vi "path_left.vi"() -> ()   [LabVIEW 2019]
uses:
  WSCbot_V3_Toolkit.lvlibp
panel:
  in  "get screw\n(XYZ) 2":cluster{"X":dbl, "Y":dbl, "Z":dbl}[](array[cluster])=[{"X"=0.0, "Y"=30.0, "Z"=0.0}, {"X"=0.0, "Y"=-30.0, "Z"=0.0}, {"X"=0.0, "Y"=0.0, "Z"=0.0}]
  in  "Stop Button 2":bool
  in  "Go home\n(XYZ)":cluster{"X":dbl, "Y":dbl, "Z":dbl}[](array[cluster])=[{"X"=0.0, "Y"=-296.0, "Z"=0.0}]
  in  "To stage\n(XYZ)":cluster{"X":dbl, "Y":dbl, "Z":dbl}[](array[cluster])=[{"X"=0.0, "Y"=-174.0, "Z"=0.0}, {"X"=143.0, "Y"=0.0, "Z"=0.0}, {"X"=0.0, "Y"=262.0, "Z"=0.0}]
  in  "get nut\nXYZ":cluster{"X":dbl, "Y":dbl, "Z":dbl}[](array[cluster])=[{"X"=0.0, "Y"=116.0, "Z"=0.0}]
  in  "cross hill\nXYZ":cluster{"X":dbl, "Y":dbl, "Z":dbl}[](array[cluster])=[{"X"=-70.0, "Y"=0.0, "Z"=0.0}, {"X"=0.0, "Y"=-145.0, "Z"=0.0}, {"X"=-77.0, "Y"=0.0, "Z"=0.0}]
  in  "to hill\n(XYZ)":cluster{"X":dbl, "Y":dbl, "Z":dbl}[](array[cluster])=[{"X"=122.0, "Y"=0.0, "Z"=0.0}, {"X"=0.0, "Y"=-60.0, "Z"=0.0}]
  in  "get screw\n(XYZ)":cluster{"X":dbl, "Y":dbl, "Z":dbl}[](array[cluster])=[{"X"=-125.0, "Y"=0.0, "Z"=0.0}, {"X"=0.0, "Y"=0.0, "Z"=0.0}, {"X"=0.0, "Y"=0.0, "Z"=0.0}]
  in  "To stage\n(XYZ)":cluster{"X":dbl, "Y":dbl, "Z":dbl}[](array[cluster])=[{"X"=66.0, "Y"=0.0, "Z"=0.0}, {"X"=0.0, "Y"=152.0, "Z"=0.0}, {"X"=70.0, "Y"=0.0, "Z"=0.0}, {"X"=0.0, "Y"=60.0, "Z"=0.0}]
  in  "To hill\n(XYZ)":cluster{"X":dbl, "Y":dbl, "Z":dbl}[](array[cluster])=[{"X"=0.0, "Y"=-106.0, "Z"=0.0}]
  in  "get nut\n(XYZ)":cluster{"X":dbl, "Y":dbl, "Z":dbl}[](array[cluster])=[{"X"=0.0, "Y"=-178.0, "Z"=-180.0}]
  in  "see mark & get screw\n(XYZ)":cluster{"X":dbl, "Y":dbl, "Z":dbl}[](array[cluster])=[{"X"=-26.0, "Y"=25.0, "Z"=0.0}, {"X"=0.0, "Y"=0.0, "Z"=-45.0}, {"X"=0.0, "Y"=0.0, "Z"=-45.0}, {"X"=0.0, "Y"=75.0, "Z"=-90.0}, {"X"=45.0, "Y"=0.0, "Z"=0.0}]
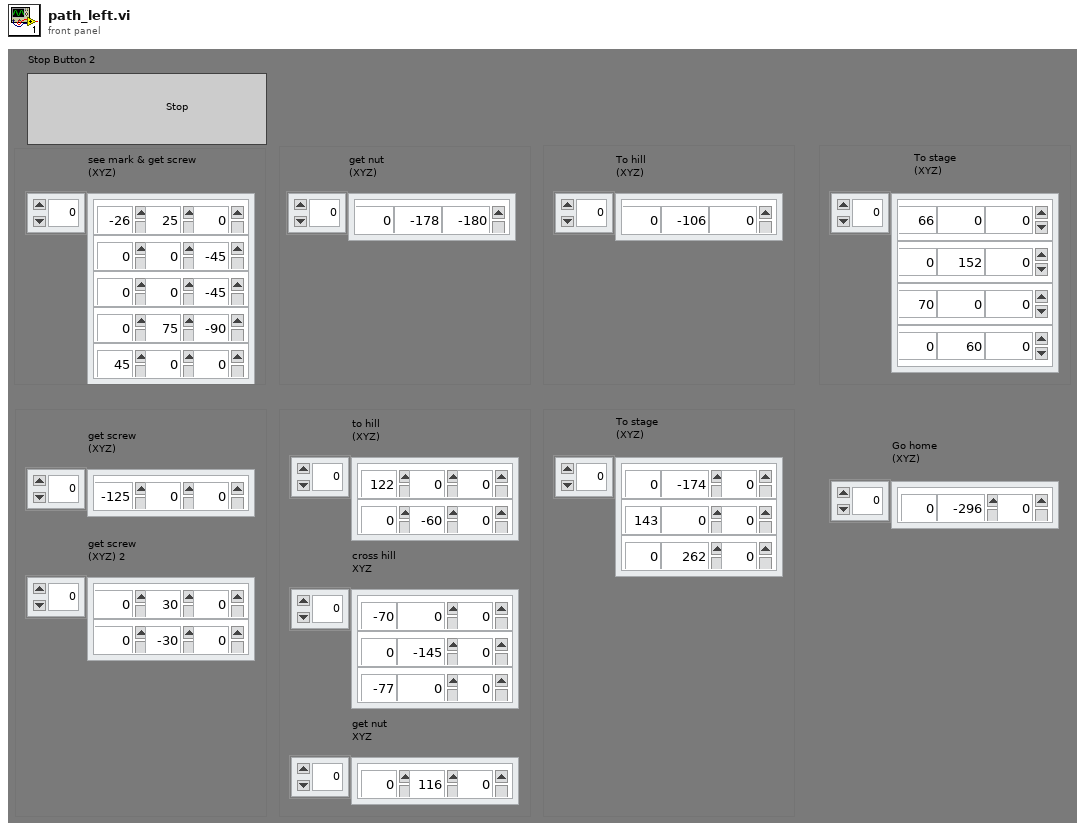
[diagram p1: front panel]
types:
  T1 = enum16{"Right_up", "Right_down", "Left_down", "Left_up", "left", "right", "up", "down"}
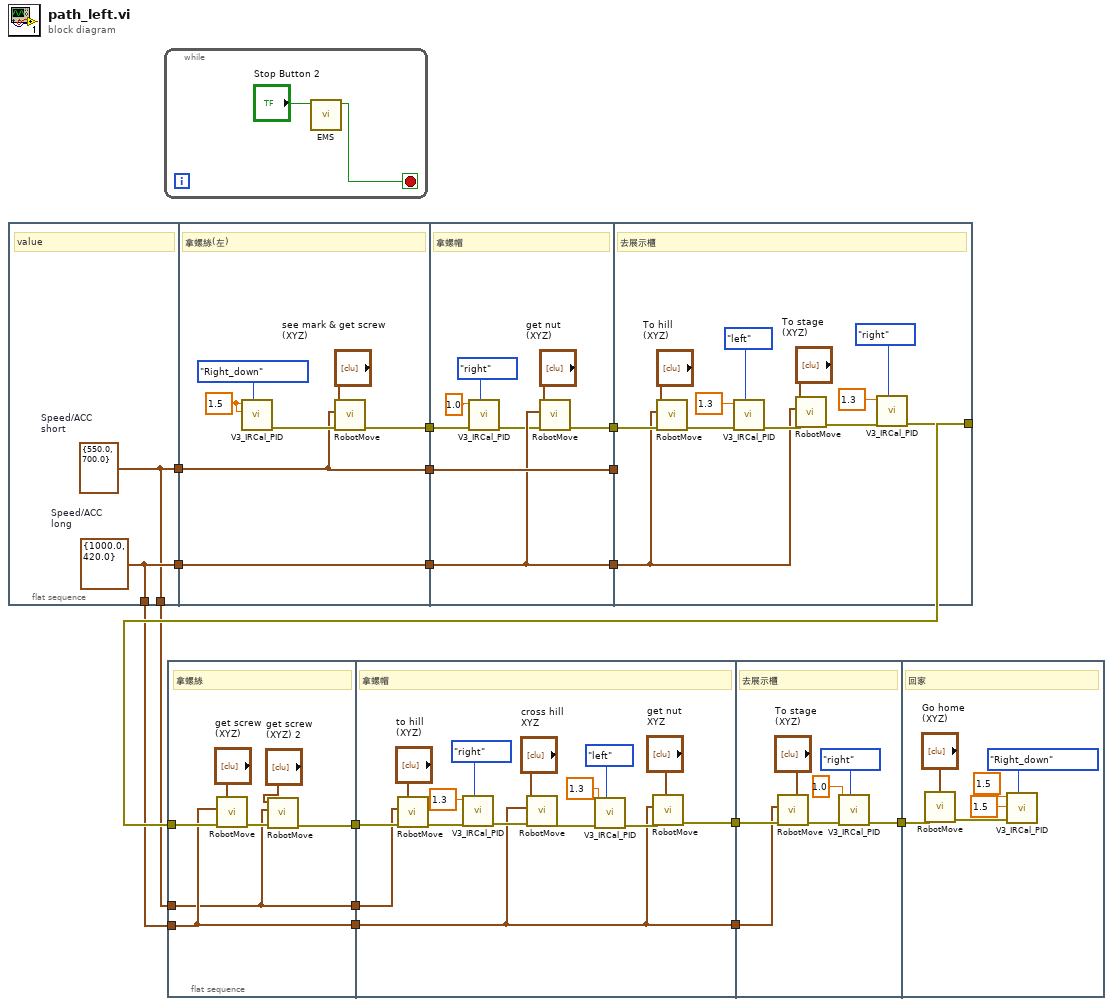
[diagram p0: block diagram]
diagram:
  n1 = flat-sequence {
    tunnel: [w18] -> w17
    tunnel: [w19] -> w10
    tunnel: [w19] -> w8
    tunnel: [w18] -> w7
    tunnel: w17 -> [w23]
    tunnel: [w24] -> w16
    tunnel: [w23] -> w14
    tunnel: [w22] -> w11
    tunnel: w10 -> [w22]
    tunnel: w16 -> [w30]
    tunnel: [w33] -> w15
    tunnel: w14 -> [w32]
    tunnel: [w32] -> w13
    tunnel: [w31] -> w12
    tunnel: w11 -> [w31]
    tunnel: w15 -> [w45]
    tunnel: w13 -> [_]
    tunnel: w12 -> [w39]
    tunnel: [w35] -> w9
    frame #0 {
      w18 = cluster{dbl, dbl} {550.0, 700.0}  # Speed/ACC short
      w19 = cluster{dbl, dbl} {1000.0, 420.0}  # Speed/ACC long
      # "value"
    }
    frame #1 {
      w21 = 1.5 ("X_distance(V)")
      # "拿螺絲(左)"
      n2 = call "V3_IRCal_PID.vi"("Direction"=T1."Right_down", "Y_distance(V)"=w21, "X_distance(V)"=w21) -> ("Error Out"=w26:errorcluster)  [unwired: 7 in, 1 out]
      n3 = call "RobotMove.vi"("error in (no error)"=w26, "Speed/ACC"=w23, "XYZ"="see mark & get screw\n(XYZ)") -> ("error out"=w24:errorcluster)  [unwired: 8 in]
    }
    frame #2 {
      # "拿螺帽"
      n4 = call "V3_IRCal_PID.vi"("Direction"=T1."right", "Error In"=w30, "X_distance(V)"=1.0) -> ("Error Out"=w29:errorcluster)  [unwired: 7 in, 1 out]
      n5 = call "RobotMove.vi"("error in (no error)"=w29, "Speed/ACC"=w31, "XYZ"="get nut\n(XYZ)") -> ("error out"=w33:errorcluster)  [unwired: 8 in]
    }
    frame #3 {
      # "去展示櫃"
      n6 = call "RobotMove.vi"("error in (no error)"=w45, "Speed/ACC"=w39, "XYZ"="To hill\n(XYZ)") -> ("error out"=w44:errorcluster)  [unwired: 8 in]
      n7 = call "V3_IRCal_PID.vi"("Direction"=T1."left", "Error In"=w44, "X_distance(V)"=1.3) -> ("Error Out"=w40:errorcluster)  [unwired: 7 in, 1 out]
      n8 = call "RobotMove.vi"("error in (no error)"=w40, "Speed/ACC"=w39, "XYZ"="To stage\n(XYZ)") -> ("error out"=w37:errorcluster)  [unwired: 8 in]
      n9 = call "V3_IRCal_PID.vi"("Direction"=T1."right", "Error In"=w37, "X_distance(V)"=1.3) -> ("Error Out"=w35:errorcluster)  [unwired: 7 in, 1 out]
    }
  }
  n10 = while {
    stop <- w47 stop-if-true
    n11 = call "EMS.vi"("ProgramStop"="Stop Button 2") -> ("EMS"=w47:bool)  [unwired: 9 in, 1 out]
  }
  n12 = flat-sequence {
    tunnel: w9 -> [w55]
    tunnel: w8 -> [w53]
    tunnel: w7 -> [w49]
    tunnel: [w51] -> w6
    tunnel: [w49] -> w5
    tunnel: [w53] -> w4
    tunnel: w6 -> [w70]
    tunnel: w5 -> [w63]
    tunnel: w4 -> [w56]
    tunnel: [w57] -> w3
    tunnel: [w56] -> w2
    tunnel: w3 -> [w76]
    tunnel: w2 -> [w72]
    tunnel: [w71] -> w1
    tunnel: w1 -> [w78]
    frame #0 {
      # "拿螺絲"
      n13 = call "RobotMove.vi"("error in (no error)"=w55, "Speed/ACC"=w53, "XYZ"="get screw\n(XYZ)") -> ("error out"=w52:errorcluster)  [unwired: 8 in]
      n14 = call "RobotMove.vi"("error in (no error)"=w52, "Speed/ACC"=w49, "XYZ"="get screw\n(XYZ) 2") -> ("error out"=w51:errorcluster)  [unwired: 8 in]
    }
    frame #1 {
      # "拿螺帽"
      n15 = call "RobotMove.vi"("error in (no error)"=w70, "Speed/ACC"=w63, "XYZ"="to hill\n(XYZ)") -> ("error out"=w68:errorcluster)  [unwired: 8 in]
      n16 = call "V3_IRCal_PID.vi"("Direction"=T1."right", "Error In"=w68, "X_distance(V)"=1.3) -> ("Error Out"=w65:errorcluster)  [unwired: 7 in, 1 out]
      n17 = call "RobotMove.vi"("error in (no error)"=w65, "Speed/ACC"=w56, "XYZ"="cross hill\nXYZ") -> ("error out"=w62:errorcluster)  [unwired: 8 in]
      n18 = call "V3_IRCal_PID.vi"("Direction"=T1."left", "Error In"=w62, "X_distance(V)"=1.3) -> ("Error Out"=w59:errorcluster)  [unwired: 7 in, 1 out]
      n19 = call "RobotMove.vi"("error in (no error)"=w59, "Speed/ACC"=w56, "XYZ"="get nut\nXYZ") -> ("error out"=w57:errorcluster)  [unwired: 8 in]
    }
    frame #2 {
      # "去展示櫃"
      n20 = call "RobotMove.vi"("error in (no error)"=w76, "Speed/ACC"=w72, "XYZ"="To stage\n(XYZ)") -> ("error out"=w75:errorcluster)  [unwired: 8 in]
      n21 = call "V3_IRCal_PID.vi"("Direction"=T1."right", "Error In"=w75, "X_distance(V)"=1.0) -> ("Error Out"=w71:errorcluster)  [unwired: 7 in, 1 out]
    }
    frame #3 {
      # "回家"
      n22 = call "RobotMove.vi"("error in (no error)"=w78, "XYZ"="Go home\n(XYZ)") -> ("error out"=w82:errorcluster)  [unwired: 9 in]
      n23 = call "V3_IRCal_PID.vi"("Direction"=T1."Right_down", "Error In"=w82, "Y_distance(V)"=1.5, "X_distance(V)"=1.5) -> ()  [unwired: 6 in, 2 out]
    }
  }
